vi "TrajectoryParam_enforceVelocity.vi"(8 "TRAJECTORY_CONFIG":T1 {"End Velocity" format="%20.4f"; "StartVelocity" format="%20.4f"; "Max Acceleration" format="%20.4f"; "MaxVelocity" format="%20.4f"}, 11 "inCONSTRAINED_STATE":T2={"POSEwCURVATURE"={"CURVATURE"=0.0, "POSE"={"TRANSLATION"={"X"=0.0, "Y"=0.0}, "ROTATION"={"VALUE"=0.0, "COS"=1.0, "SIN"=0.0}}}, "Distance"=0.0, "minAccel"=0.0, "maxAccel"=0.0, "maxVelocity"=0.0} {"POSEwCURVATURE"."POSE"."ROTATION"."SIN" format="%13.4f"; "POSEwCURVATURE"."POSE"."ROTATION"."COS" format="%13.4f"; "POSEwCURVATURE"."POSE"."ROTATION"."VALUE" format="%13.4f"; "POSEwCURVATURE"."POSE"."TRANSLATION"."Y" format="%14.3f"; "POSEwCURVATURE"."POSE"."TRANSLATION"."X" format="%14.3f"}) -> (0 "error out":errorcluster, 3 "outCONSTRAINED_STATE":T2={"POSEwCURVATURE"={"CURVATURE"=0.0, "POSE"={"TRANSLATION"={"X"=0.0, "Y"=0.0}, "ROTATION"={"VALUE"=0.0, "COS"=1.0, "SIN"=0.0}}}, "Distance"=0.0, "minAccel"=0.0, "maxAccel"=0.0, "maxVelocity"=0.0} {"POSEwCURVATURE"."POSE"."ROTATION"."SIN" format="%13.4f"; "POSEwCURVATURE"."POSE"."ROTATION"."COS" format="%13.4f"; "POSEwCURVATURE"."POSE"."ROTATION"."VALUE" format="%13.4f"; "POSEwCURVATURE"."POSE"."TRANSLATION"."Y" format="%14.3f"; "POSEwCURVATURE"."POSE"."TRANSLATION"."X" format="%14.3f"})   [LabVIEW 2019, in "Trajectory_Library.lvlib"]
doc: "Internal routine called by TrajectoryParam_timeParam.VI \n\nThis routine enforces velocity constraints and updates the ConstrainedState value based on the calculated limits.\n\nThis routine will need to be updated whenever a new constrained state type is added.\n------------------------------------------------------------------------------------------\n\nParameters:\n - InConstrainedState\n - TrajectoryConfig\n\nReturns\n - OutConstrainedState\n - error out"
uses:
  Trajectory_Library.lvlib
  <vilib>/Utility/Data Type/NI_Data Type.lvlib
  TypeDef/DIFF_DRIVE_KINEMATICS.ctl
  TypeDef/TRAJ_CONSTRAINT_DIIF_DRIVE_KINEMATICS.ctl
  TypeDef/TRAJ_CONSTRAINT_CENTRIPETAL_ACCEL.ctl
  TypeDef/SIMPLE_MOTOR_FF.ctl
  TypeDef/TRAJ_CONSTRAINT_DIIF_DRIVE_VOLTAGE.ctl
  TypeDef/TRANSLATION2D.ctl
  <vilib>/Analysis/Matrix/Datatypes/RealMatrix.ctl
  <vilib>/Analysis/Matrix/NI_Matrix.lvlib
  TypeDef/MECA_DRIVE_KINEMATICS.ctl
  TypeDef/TRAJ_CONSTRAINT_MECA_DRIVE_KINEMATICS.ctl
  TypeDef/SWERVE_DRIVE_KINEMATICS.ctl
  TypeDef/TRAJ_CONSTRAINT_SWERVE_DRIVE_KINEMATICS.ctl
  TypeDef/TRAJ_CONSTRAINT_MAX_VELOCITY.ctl
  Enum/TRAJ_CONSTRAINT_TYPES_ENUM.ctl
  TypeDef/TRAJ_CONSTRAINT_ELLIP_REGION.ctl
  TypeDef/TRAJ_CONSTRAINT_RECT_REGION.ctl
  TypeDef/ROTATION2D.ctl
  TypeDef/SWERVE_DRIVE_MODULE_STATE.ctl
  TypeDef/POSE2D.ctl
  TypeDef/POSEwCURVATURE.ctl
  TypeDef/CONSTRAINED_STATE.ctl
  TypeDef/TRAJ_CONFIG.ctl
panel:
  # "All units\nare SI"
  # "All units\nare SI"
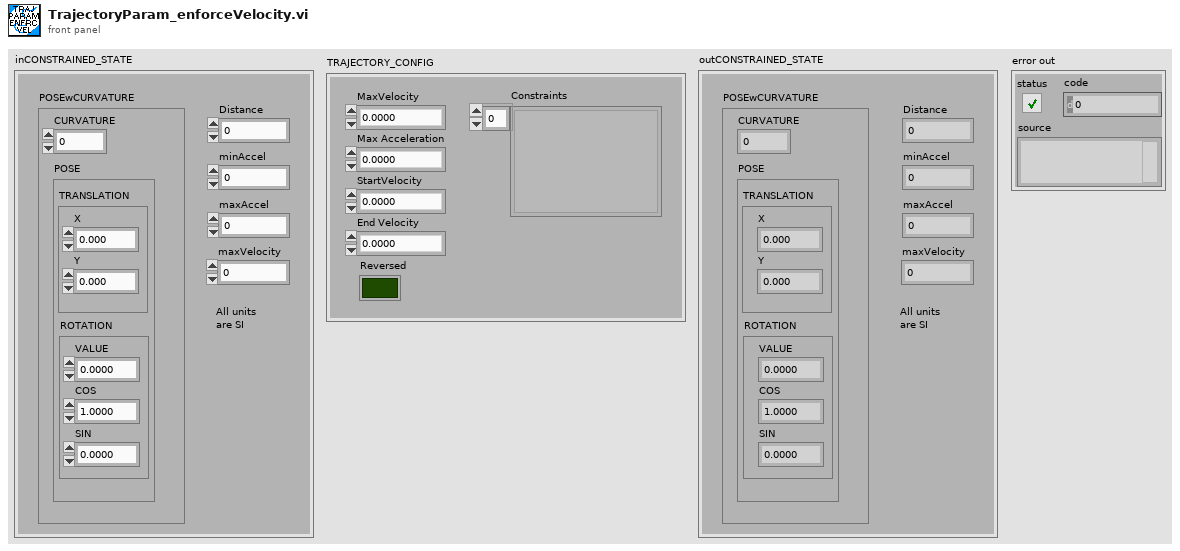
[diagram p1: front panel]
types:
  T1 = typedef "Trajectory_Library.lvlib/TRAJ_CONFIG.ctl" = cluster{"MaxVelocity":dbl, "Max Acceleration":dbl, "StartVelocity":dbl, "End Velocity":dbl, "Reversed":bool, "Constraints":variant[]}
  T2 = typedef "Trajectory_Library.lvlib/CONSTRAINED_STATE.ctl" = cluster{"POSEwCURVATURE":T3, "Distance":dbl, "minAccel":dbl, "maxAccel":dbl, "maxVelocity":dbl}
  T3 = typedef "Trajectory_Library.lvlib/POSEwCURVATURE.ctl" = cluster{"CURVATURE":dbl, "POSE":T4}
  T4 = typedef "Trajectory_Library.lvlib/POSE2D.ctl" = cluster{"TRANSLATION":T5, "ROTATION":T6}
  T5 = typedef "Trajectory_Library.lvlib/TRANSLATION2D.ctl" = cluster{"X":dbl, "Y":dbl}
  T6 = typedef "Trajectory_Library.lvlib/ROTATION2D.ctl" = cluster{"VALUE":dbl, "COS":dbl, "SIN":dbl}
  T7 = typedef "Trajectory_Library.lvlib/TRAJ_CONSTRAINT_DIIF_DRIVE_KINEMATICS.ctl" = cluster{"Max Speed (M/S)":dbl, "DIFF_DRIVE_KINEMATICS":T8, "Max Accel (M/S2)":dbl}
  T8 = typedef "Trajectory_Library.lvlib/DIFF_DRIVE_KINEMATICS.ctl" = cluster{"TrackWidth_Meters":dbl}
  T9 = typedef "Trajectory_Library.lvlib/TRAJ_CONSTRAINT_CENTRIPETAL_ACCEL.ctl" = cluster{"Max Cent Accel":dbl}
  T10 = typedef "Trajectory_Library.lvlib/TRAJ_CONSTRAINT_DIIF_DRIVE_VOLTAGE.ctl" = cluster{"Max Voltage":dbl, "DIFF_DRIVE_KINEMATICS":T8, "SIMPLE_MOTOR_FF":T11}
  T11 = typedef "Trajectory_Library.lvlib/SIMPLE_MOTOR_FF.ctl" = cluster{"Ks":dbl, "Kv":dbl, "Ka":dbl, "KnInv":dbl}
  T12 = typedef "Trajectory_Library.lvlib/TRAJ_CONSTRAINT_MECA_DRIVE_KINEMATICS.ctl" = cluster{"Max Speed (M/S)":dbl, "MECA_DRIVE_KINEMATICS":T13}
  T13 = typedef "Trajectory_Library.lvlib/MECA_DRIVE_KINEMATICS.ctl" = cluster{"FrontLeft":T5, "FrontRight":T5, "RearLeft":T5, "RearRight":T5, "InverseKinematics":T14, "ForwardKinematics":T14, "PrevCoR":T5}
  T14 = typedef "NI_Matrix.lvlib/RealMatrix.ctl" = dbl[][]
  T15 = typedef "Trajectory_Library.lvlib/TRAJ_CONSTRAINT_SWERVE_DRIVE_KINEMATICS.ctl" = cluster{"Max Speed (M/S)":dbl, "SwerveKinematics":T16}
  T16 = typedef "Trajectory_Library.lvlib/SWERVE_DRIVE_KINEMATICS.ctl" = cluster{"NumModules":i32, "InverseKinematics":T14, "ForwardKinematics":T14, "Modules":T5[], "PrevCoR":T5, "SavedModuleStates":T17[]}
  T17 = typedef "Trajectory_Library.lvlib/SWERVE_DRIVE_MODULE_STATE.ctl" = cluster{"Speed":dbl, "Angle":T6}
  T18 = typedef "Trajectory_Library.lvlib/TRAJ_CONSTRAINT_MAX_VELOCITY.ctl" = cluster{"Max Velocity":dbl, "IM UNIQUE":bool}
  T19 = typedef "Trajectory_Library.lvlib/TRAJ_CONSTRAINT_ELLIP_REGION.ctl" = cluster{"Center":T5, "Radii":T5, "Constraint":variant, "Constraint Type":T20, "IM UNIQUE":bool}
  T20 = typedef "Trajectory_Library.lvlib/TRAJ_CONSTRAINT_TYPES_ENUM.ctl" = enum16{"UNDEFINED", "DIFF DRIVE KINEMATICS", "DIFF DRIVE VOLTAGE", "CENTRIPITAL ACCEL", "MECA DRIVE KINEMATICS", "SWERVE DRIVE KINEMATICS", "MAXIMUM VELOCITY", "ELLIPTICAL REGION", "RECTANGULAR REGION"}
  T21 = typedef "Trajectory_Library.lvlib/TRAJ_CONSTRAINT_RECT_REGION.ctl" = cluster{"BottomLeftPoint":T5, "TopRightPoint":T5, "Constraint":variant, "Constraint Type":T20}
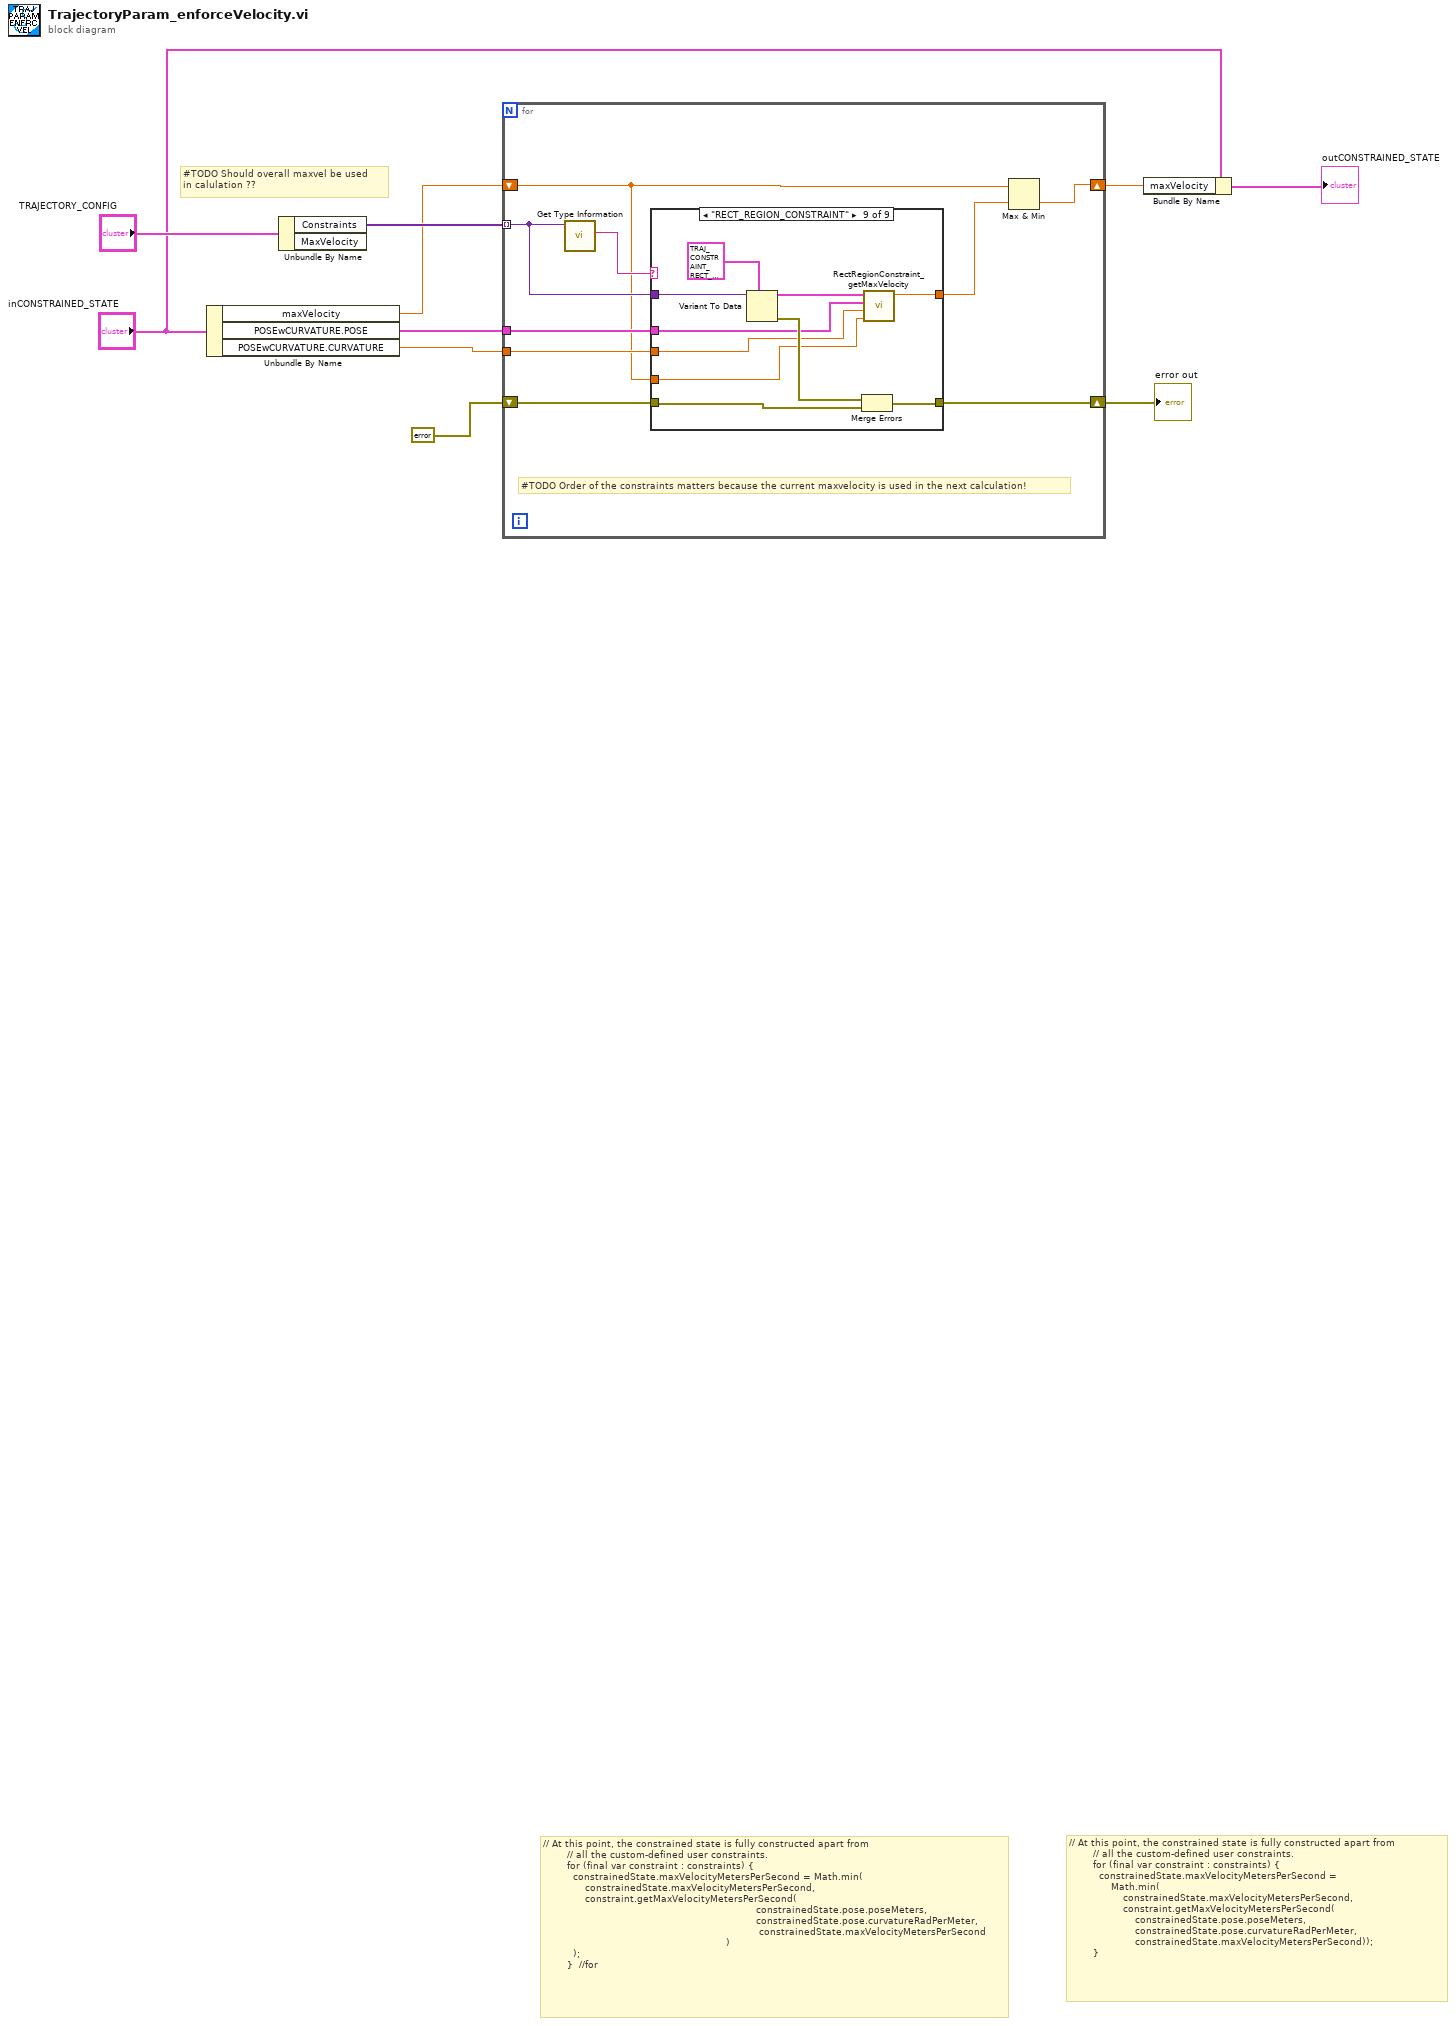
[diagram p0: block diagram]
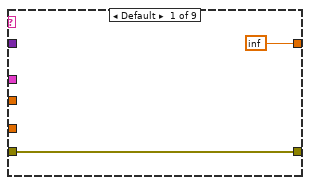
[diagram p2: hidden frame]
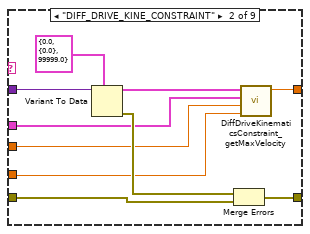
[diagram p3: hidden frame]
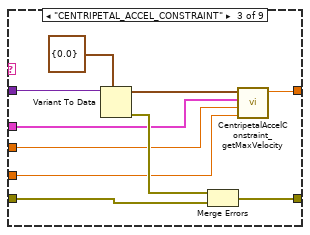
[diagram p4: hidden frame]
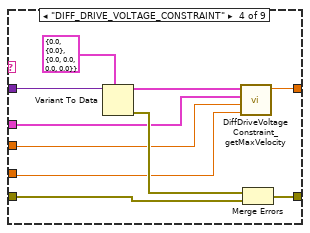
[diagram p5: hidden frame]
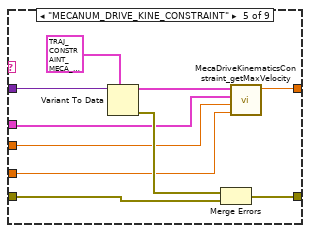
[diagram p6: hidden frame]
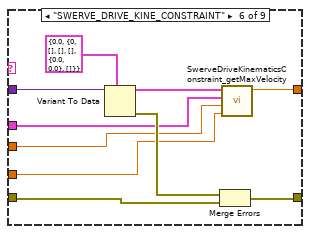
[diagram p7: hidden frame]
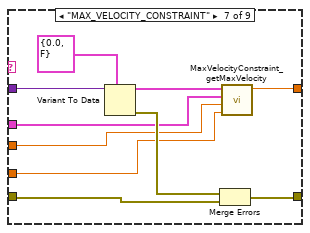
[diagram p8: hidden frame]
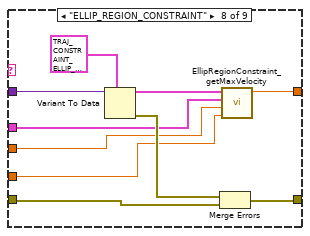
[diagram p9: hidden frame]
diagram:
  # "#TODO Should overall maxvel be used\nin calulation ??"
  # "// At this point, the constrained state is fully constructed apart from\n        // all the custom-defined user constraints.\n        for (final var constraint : constraints) {\n          constrainedState.maxVelocityMetersPerSecond =\n              Math.min(\n                  constrainedState.maxVelocityMetersPerSecond,\n                  constraint.getMaxVelocityMetersPerSecond(\n                      constrainedState.pose.poseMeters,\n                      constrainedState.pose.curvatureRadPerMeter,\n                      constrainedState.maxVelocityMetersPerSecond));\n        }"
  # "// At this point, the constrained state is fully constructed apart from\n        // all the custom-defined user constraints.\n        for (final var constraint : constraints) {\n          constrainedState.maxVelocityMetersPerSecond = Math.min(\n              constrainedState.maxVelocityMetersPerSecond,\n              constraint.getMaxVelocityMetersPerSecond(\n                                                                       constrainedState.pose.poseMeters, \n                                                                       constrainedState.pose.curvatureRadPerMeter,\n                                                                        constrainedState.maxVelocityMetersPerSecond\n                                                             )\n          );\n        }  //for"
  n1 = Unbundle By Name("inCONSTRAINED_STATE") -> ("maxVelocity"=w2:dbl, "POSEwCURVATURE.POSE"=w6:T4, "POSEwCURVATURE.CURVATURE"=w5:dbl)
  n2 = Unbundle By Name("TRAJECTORY_CONFIG") -> ("Constraints"=w4:variant[])  [unwired: 1 out]
  n3 = for {
    tunnel: w4 -> [w18] mode=indexing
    tunnel: w6 -> [w17]
    tunnel: w5 -> [w16]
    shift-right: [w15] -> w3
    shift-left: errorcluster {"status"=FALSE, "code"=0, "source"=""} ("error IO") -> [w14]
    shift-right: [w13] -> w1
    shift-left: w2 -> [w11]
    # "#TODO Order of the constraints matters because the current maxvelocity is used in the next calculation!"
    n4 = call <vilib>:"Get Type Information.vi"("variant"=w18) -> ("name"=w19:string)  [unwired: 6 in, 4 out]
    n5 = case shown="\"RECT_REGION_CONSTRAINT\"" w19 {
      tunnel: w18 -> [_ w31 w41 w51 w61 w71 w81 w91 w101]
      tunnel: w17 -> [_ w25 w35 w45 w55 w65 w75 w85 w95]
      tunnel: w16 -> [_ w24 w34 w44 w54 w64 w74 w84 w94]
      tunnel: w11 -> [_ w23 w33 w43 w53 w63 w73 w83 w93]
      tunnel: [w21 w29 w40 w49 w60 w70 w80 w90 w100] -> w15
      tunnel: w14 -> [w21 w28 w38 w48 w58 w68 w78 w88 w98]
      tunnel: [inf w22 w32 w42 w52 w62 w72 w82 w92] -> w12
      frame Default {
      }
      frame "DIFF_DRIVE_KINE_CONSTRAINT" {
        n6 = Variant To Data(type=T7 {"Max Speed (M/S)"=0.0, "DIFF_DRIVE_KINEMATICS"={"TrackWidth_Meters"=0.0}, "Max Accel (M/S2)"=99999.0} ("DIFF_DRIVE_KINE_CONSTRAINT"), Variant=w31) -> (data=w26:T7, error out=w30:errorcluster)  [unwired: 1 in]
        n7 = Merge Errors(w30, w28) -> (w29:errorcluster)
        n8 = call "DiffDriveKinematicsConstraint_getMaxVelocity.vi"("Velocity"=w23, "Curvature"=w24, "statePose"=w25, "DIFF_DRIVE_KINE_CONSTRAINT"=w26) -> ("absMaxVelocity"=w22:dbl)  [unwired: 7 in]
      }
      frame "CENTRIPETAL_ACCEL_CONSTRAINT" {
        n9 = Variant To Data(type=T9 {"Max Cent Accel"=0.0} ("CENTRIPETAL_ACCEL_CONSTRAINT"), Variant=w41) -> (data=w36:T9, error out=w39:errorcluster)  [unwired: 1 in]
        n10 = Merge Errors(w39, w38) -> (w40:errorcluster)
        n11 = call "CentripetalAccelConstraint_getMaxVelocity.vi"("Velocity"=w33, "Curvature"=w34, "statePose"=w35, "CENTRIPETAL_ACCEL_CONSTRAINT"=w36) -> ("absMaxVelocity"=w32:dbl)  [unwired: 7 in]
      }
      frame "DIFF_DRIVE_VOLTAGE_CONSTRAINT" {
        n12 = Variant To Data(type=T10 {"Max Voltage"=0.0, "DIFF_DRIVE_KINEMATICS"={"TrackWidth_Meters"=0.0}, "SIMPLE_MOTOR_FF"={"Ks"=0.0, "Kv"=0.0, "Ka"=0.0, "KnInv"=0.0}} ("DIFF_DRIVE_VOLTAGE_CONSTRAINT"), Variant=w51) -> (data=w46:T10, error out=w50:errorcluster)  [unwired: 1 in]
        n13 = call "DiffDriveVoltageConstraint_getMaxVelocity.vi"("Velocity"=w43, "Curvature"=w44, "statePose"=w45, "DIFF_DRIVE_VOLTAGE_CONSTRAINT"=w46) -> ("absMaxVelocity"=w42:dbl)  [unwired: 7 in]
        n14 = Merge Errors(w50, w48) -> (w49:errorcluster)
      }
      frame "MECANUM_DRIVE_KINE_CONSTRAINT" {
        n15 = Variant To Data(type=T12 {"Max Speed (M/S)"=0.0, "MECA_DRIVE_KINEMATICS"={"FrontLeft"={"X"=0.0, "Y"=0.0}, "FrontRight"={"X"=0.0, "Y"=0.0}, "RearLeft"={"X"=0.0, "Y"=0.0}, "RearRight"={"X"=0.0, "Y"=0.0}, "InverseKinematics"=[[0.0, 1.0, -1.0, 0.0], [0.0, 1.0, 1.0, 0.0], [0.0, 1.0, 1.0, 0.0], [0.0, 1.0, -1.0, 0.0]], "ForwardKinematics"=[[0.0, 1.0, -1.0, 0.0], [0.0, 1.0, 1.0, 0.0], [0.0, 1.0, 1.0, 0.0], [0.0, 1.0, -1.0, 0.0]], "PrevCoR"={"X"=0.0, "Y"=0.0}}} ("MECANUM_DRIVE_KINE_CONSTRAINT"), Variant=w61) -> (data=w56:T12, error out=w59:errorcluster)  [unwired: 1 in]
        n16 = Merge Errors(w59, w58) -> (w60:errorcluster)
        n17 = call "MecaDriveKinematicsConstraint_getMaxVelocity.vi"("Velocity"=w53, "Curvature"=w54, "statePose"=w55, "MECANUM_DRIVE_KINE_CONSTRAINT"=w56) -> ("absMaxVelocity"=w52:dbl)  [unwired: 7 in]
      }
      frame "SWERVE_DRIVE_KINE_CONSTRAINT" {
        n18 = Variant To Data(type=T15 {"Max Speed (M/S)"=0.0, "SwerveKinematics"={"NumModules"=0, "InverseKinematics"=[], "ForwardKinematics"=[], "Modules"=[], "PrevCoR"={"X"=0.0, "Y"=0.0}, "SavedModuleStates"=[]}} ("SWERVE_DRIVE_KINE_CONSTRAINT"), Variant=w71) -> (data=w66:T15, error out=w69:errorcluster)  [unwired: 1 in]
        n19 = Merge Errors(w69, w68) -> (w70:errorcluster)
        n20 = call "SwerveDriveKinematicsConstraint_getMaxVelocity.vi"("Velocity"=w63, "Curvature"=w64, "statePose"=w65, "SWERVE_DRIVE_KINE_CONSTRAINT"=w66) -> ("absMaxVelocity"=w62:dbl)  [unwired: 7 in]
      }
      frame "MAX_VELOCITY_CONSTRAINT" {
        n21 = Variant To Data(type=T18 {"Max Velocity"=0.0, "IM UNIQUE"=FALSE} ("MAX_VELOCITY_CONSTRAINT"), Variant=w81) -> (data=w76:T18, error out=w79:errorcluster)  [unwired: 1 in]
        n22 = Merge Errors(w79, w78) -> (w80:errorcluster)
        n23 = call "MaxVelocityConstraint_getMaxVelocity.vi"("Velocity"=w73, "Curvature"=w74, "statePose"=w75, "MAX_VELOCITY_CONSTRAINT"=w76) -> ("absMaxVelocity"=w72:dbl)  [unwired: 7 in]
      }
      frame "ELLIP_REGION_CONSTRAINT" {
        n24 = Variant To Data(type=T19 {"Center"={"X"=0.0, "Y"=0.0}, "Radii"={"X"=0.0, "Y"=0.0}, "Constraint"=variant, "Constraint Type"=enum."DIFF DRIVE KINEMATICS", "IM UNIQUE"=FALSE} ("ELLIP_REGION_CONSTRAINT"), Variant=w91) -> (data=w86:T19, error out=w89:errorcluster)  [unwired: 1 in]
        n25 = Merge Errors(w89, w88) -> (w90:errorcluster)
        n26 = call "EllipRegionConstraint_getMaxVelocity.vi"("Velocity"=w83, "Curvature"=w84, "statePose"=w85, "ELLIP_REGION_CONSTRAINT"=w86) -> ("absMaxVelocity"=w82:dbl)  [unwired: 7 in]
      }
      frame "RECT_REGION_CONSTRAINT" {
        n27 = Variant To Data(type=T21 {"BottomLeftPoint"={"X"=0.0, "Y"=0.0}, "TopRightPoint"={"X"=0.0, "Y"=0.0}, "Constraint"=variant, "Constraint Type"=enum."DIFF DRIVE KINEMATICS"} ("RECT_REGION_CONSTRAINT"), Variant=w101) -> (data=w96:T21, error out=w99:errorcluster)  [unwired: 1 in]
        n28 = Merge Errors(w99, w98) -> (w100:errorcluster)
        n29 = call "RectRegionConstraint_getMaxVelocity.vi"("Velocity"=w93, "Curvature"=w94, "statePose"=w95, "RECT_REGION_CONSTRAINT"=w96) -> ("absMaxVelocity"=w92:dbl)  [unwired: 7 in]
      }
    }
    n30 = Max & Min(x=w11, y=w12) -> (min(x,y)=w13:dbl)  [unwired: 1 out]
  }
  "error out" <- w3
  n31 = Bundle By Name(cluster="inCONSTRAINED_STATE", "maxVelocity"=w1) -> (→"outCONSTRAINED_STATE":T2)
